vi "LibXML_ReplaceNodeContent.vi"(8 "error in":errorcluster, 9 "New Value":string, 10 "xpathexpr":string="/ScanMaster/Devices/Device/description", 11 "doc":u32) -> (0 "error out":errorcluster, 3 "doc copy out":u32)   [LabVIEW 2019, in "Tools.lvlib" / "LibXML.lvlib"]
uses:
  LibXML.lvlib
  Error Cluster From Error Code_subroutine.vi
  <vilib>/Utility/error.llb/Trim Whitespace.vi
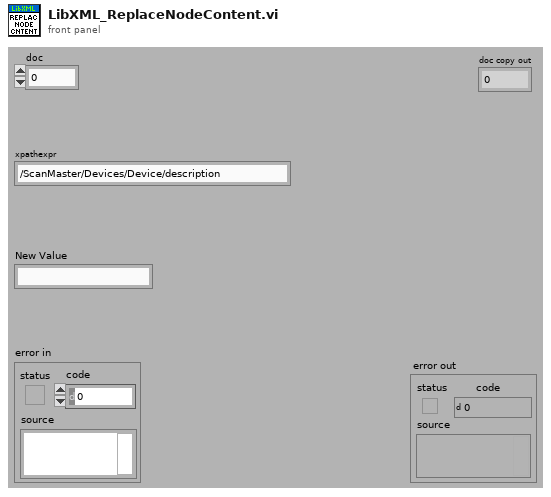
[diagram p1: front panel]
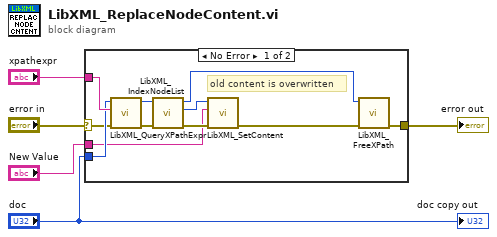
[diagram p0: block diagram]
diagram:
  n1 = case shown="No Error" "error in" {
    selector: "error in" -> [w6 w17]
    tunnel: "xpathexpr" -> [w16 _]
    tunnel: "doc" -> [w15 _]
    tunnel: [w14 w17] -> w3
    tunnel: "New Value" -> [w7 _]
    frame No Error {
      # "old content is overwritten"
      n2 = call "LibXML_QueryXPathExpr.vi"("error in"=w6, "XPathExpr"=w16, "doc"=w15) -> ("error out"=w12:errorcluster, "xmlXPathObj"=w13:u32)  [unwired: 7 in]
      n3 = call "LibXML_IndexNodeList.vi"("error in"=w12, "XPathObj"=w13) -> ("error out"=w11:errorcluster, "NodePtr"=w8:u32, "XPathObj out"=w9:u32)  [unwired: 7 in]
      n4 = call "LibXML_SetContent.vi"("error in (no error)"=w11, "content"=w7, "node"=w8) -> ("error out"=w10:errorcluster)  [unwired: 7 in, 1 out]
      n5 = call "LibXML_FreeXPath.vi"("error in"=w10, "XPathObj"=w9) -> ("error out"=w14:errorcluster)  [unwired: 9 in]
    }
    frame Error {
    }
  }
  "error out" <- w3
  "doc copy out" <- "doc"
